vi "MEASURE_hysteresis_multiple_gate_Raman - set voltage.vi"() -> ()   [LabVIEW 2020]
uses:
  <instrlib>/Keithley 24XX/Public/Data/Read (Multiple Points).vi
  <vilib>/Utility/file.llb/Write To Spreadsheet File (DBL).vi
  <instrlib>/Stanford Research 830/Stanford Research 830.lvlib
  <instrlib>/Keithley 24XX/Keithley 24XX.lvlib
  <instrlib>/Keithley 2450/Keithley 2450.lvlib
  <vilib>/Analysis/NI_AALBase.lvlib
panel:
  in  "GATE final Value":dbl=6.0
  in  "Gate sequence":dbl
  out "while loop":dbl
  in  "topgate-off set":dbl=-5.0
  in  "0ff set{T}/no off set[F]":bool
  out "XY Graph 4":cluster{dbl[], dbl[]}(graph)
  out "XY Graph 3":cluster{dbl[], dbl[]}(graph)
  out "top gate leaking":dbl=2.469318360898143e-10
  out "bottom gate voltage":dbl format="%#_13g"
  in  "Compliance  Level (1uA)":dbl=1.9999999995789155e-07
  in  "Source Mode  (0: Voltage)":u16(ring) items=["Voltage", "Current"]
  in  "Serial Configuration":T1={"Baud Rate"=9600, "Parity"=0, "Data Bits"=8, "Stop Bits"=10, "Flow Control"=0} {"Flow Control" items=["None", "XON/XOFF", "RTS/CTS", "XON/XOFF & RTS/CTS", "DTR/DSR", "XON/XOFF & DTR/DSR"]; "Stop Bits" items=["1.0"=10, "1.5"=15, "2.0"=20]; "Data Bits" items=["7"=7, "8"=8]; "Parity" items=["None", "Odd", "Even", "Mark", "Space"]; "Baud Rate" items=["300"=300, "600"=600, "1200"=1200, "2400"=2400, "4800"=4800, "9600"=9600, "19200"=19200]}
  in  "backgate address":refnum<visa-resource-name>="GPIB0::25::INSTR"
  in  "bottom gate thickness":dbl=10.0
  in  "top gate thickness":dbl=30.0
  in  "pure field (T)/pure doping (F)":bool
  out "loop run":i32=2
  in  "loop #":i32=2
  in  "Save data or not":bool=TRUE
  in  "path (folder + filename)":string="C:\\Users\\User\\Data\\Jason\\03282019\\ pure_bottom_high_6v_rato3 with light2"
  in  "Clear Plot":bool
  out "LOCKIN Measurement":dbl=0.9110010000000001
  in  "Parameter (1: X)":u16(ring)=1 items=["X"=1, "Y"=2, "R"=3, "Theta"=4, "Channel 1"=5, "Channel 2"=6, "Aux In 1"=7, "Aux In 2"=8, "Aux In 3"=9, "Aux In 4"=10]
  out "top gate voltage":dbl format="%#_13g"
  out "back gate leaking":string="-9.306248E-12\n"
  in  "GATE STEP(mv)":i32=450
  in  "GATE Low Value (default 0)":dbl
  in  "GATE High Value":dbl=18.0
  in  "Function (0: Volts) 2":u16(ring) items=["Volts", "Current", "Resistance"]
  in  "Source Compaliance":dbl=1.000000000000001e-07
  in  "topgate address":refnum<visa-resource-name>="GPIB0::18::INSTR"
  in  "SD stabilization(S) 2":dbl=0.1 format="%#_13g"
  in  "Sine Output Amplitude (1 V) 2":dbl=0.05
  in  "GATE / SD stablization 3":dbl=0.1 format="%#_13g"
  in  "frequency":dbl=50.0 format="%#_13g"
  in  "Input Connection (0: Single-Ended Voltage)":u16(ring) items=["Single-Ended Voltage", "Differential Voltage", "1 MOhm Current Gain", "100 MOhm Current Gain"]
  in  "LOCKIN address":refnum<visa-resource-name>="GPIB0::8::INSTR"
  # "Gate2401(back) Setting"
  # "Lock-in"
  # "Gate2450(top) Setting"
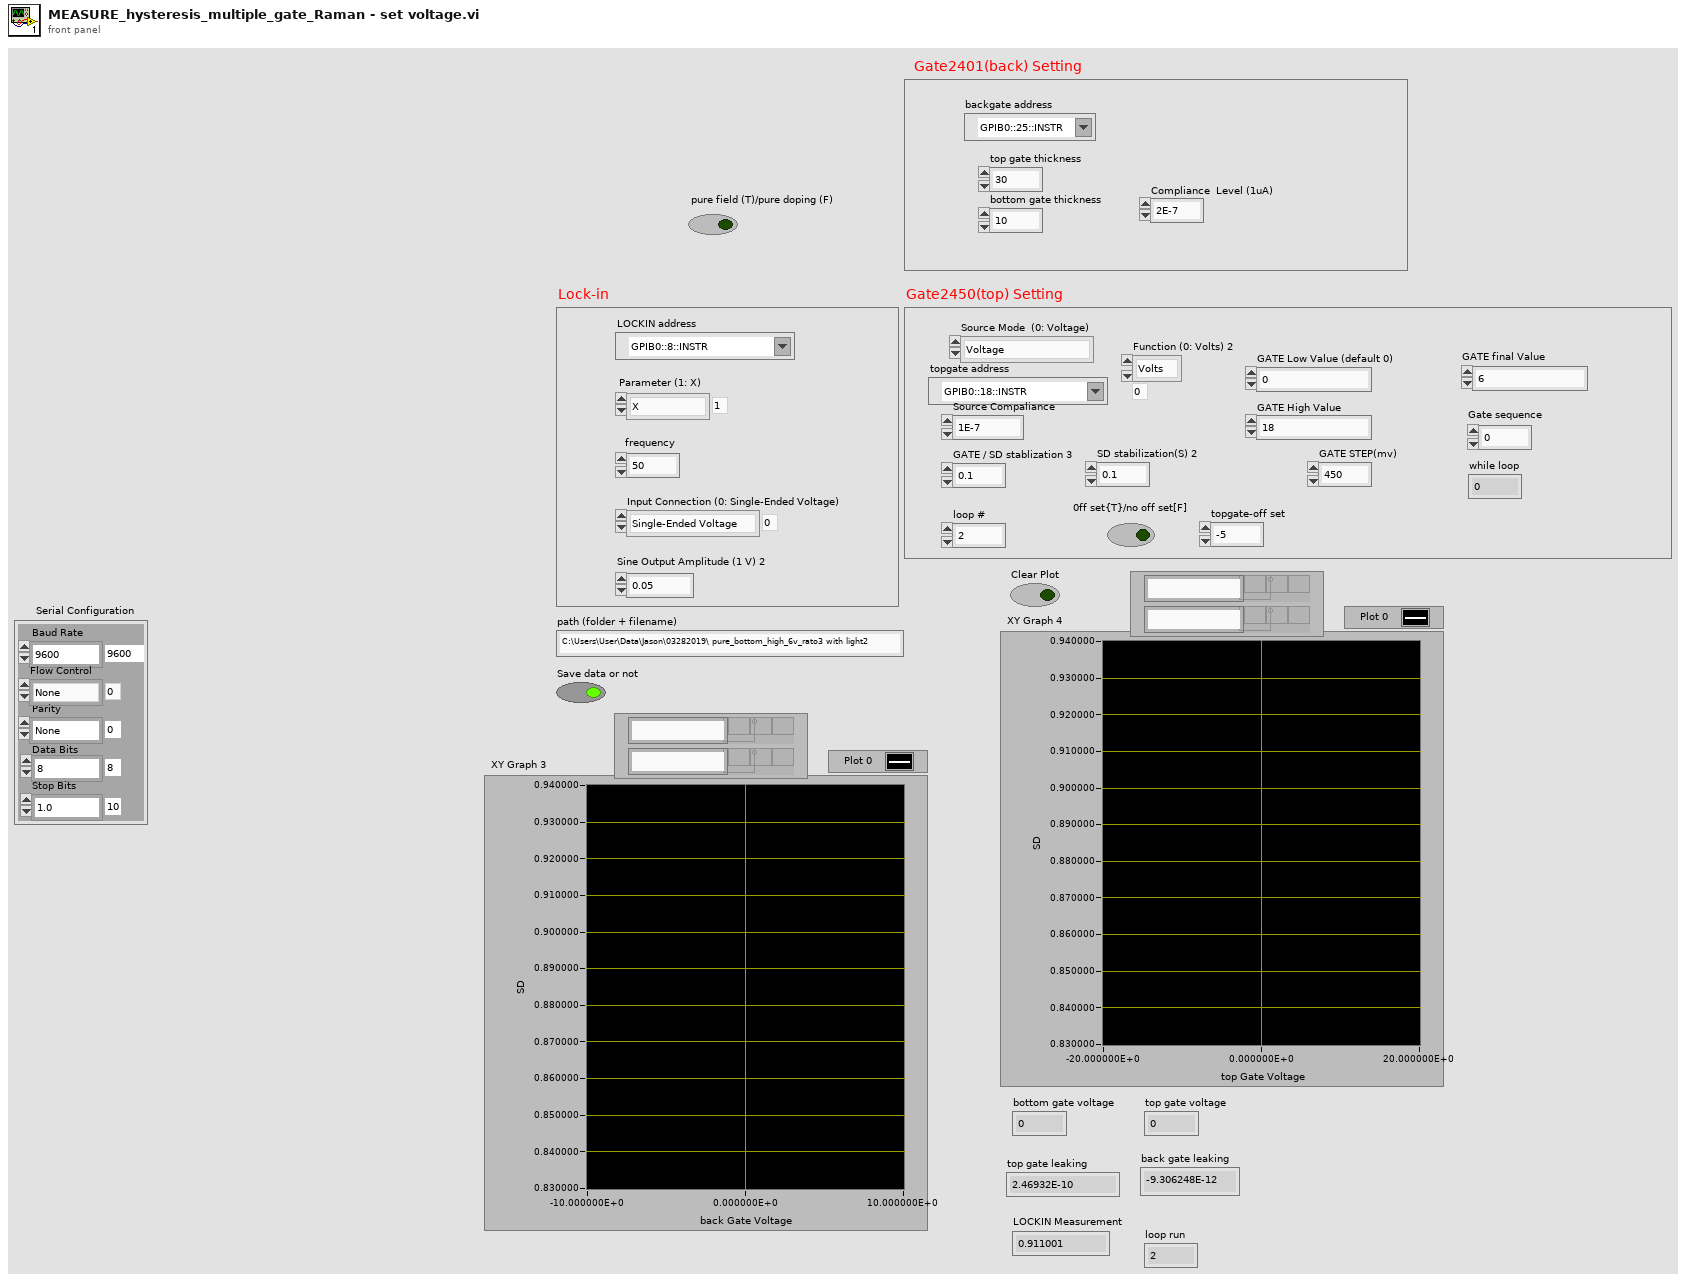
[diagram p1: front panel]
types:
  T1 = cluster{"Baud Rate":u32, "Parity":u16, "Data Bits":u16, "Stop Bits":u16, "Flow Control":u16}
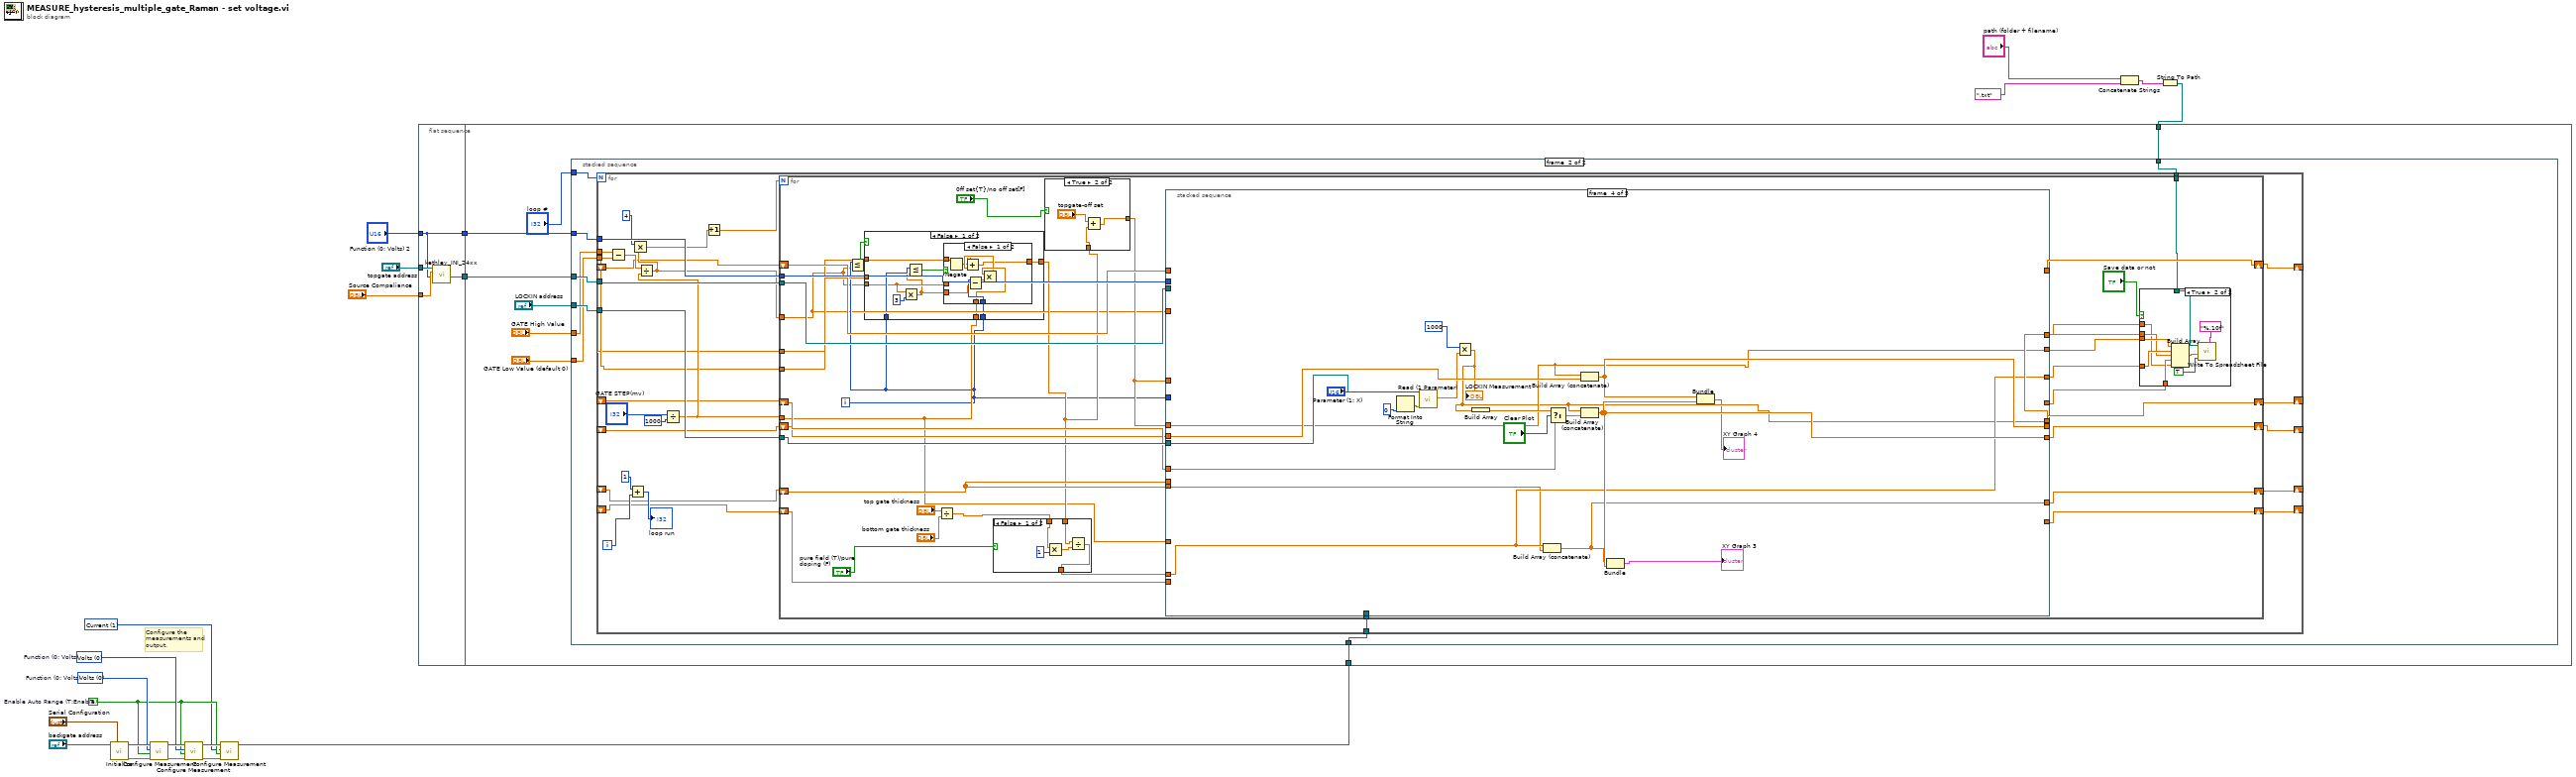
[diagram p0: block diagram]
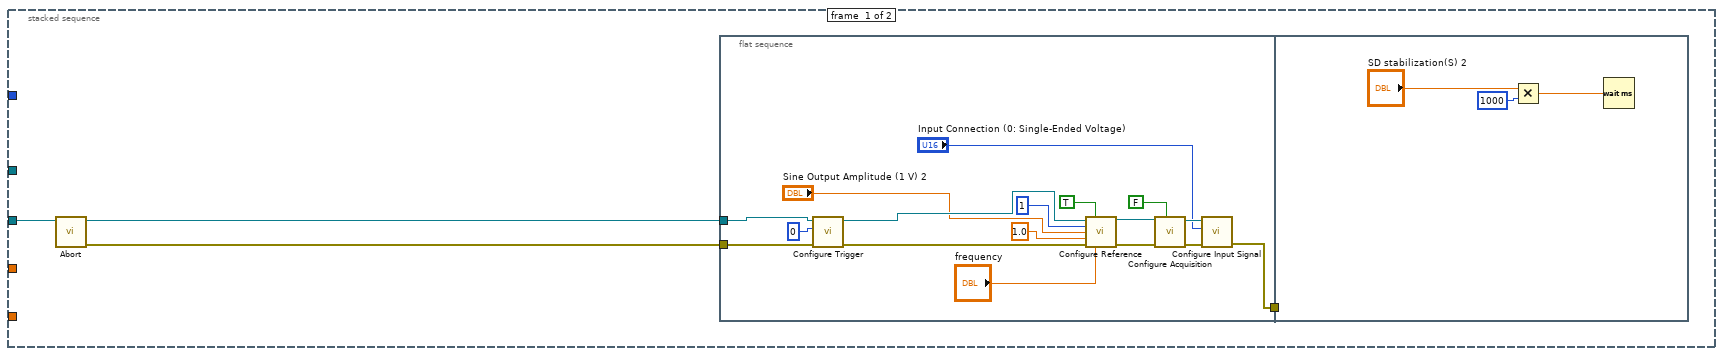
[diagram p2: hidden frame]
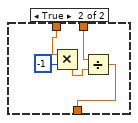
[diagram p4: hidden frame]
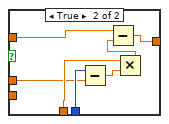
[diagram p6: hidden frame]
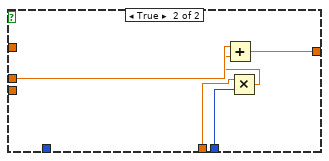
[diagram p7: hidden frame]
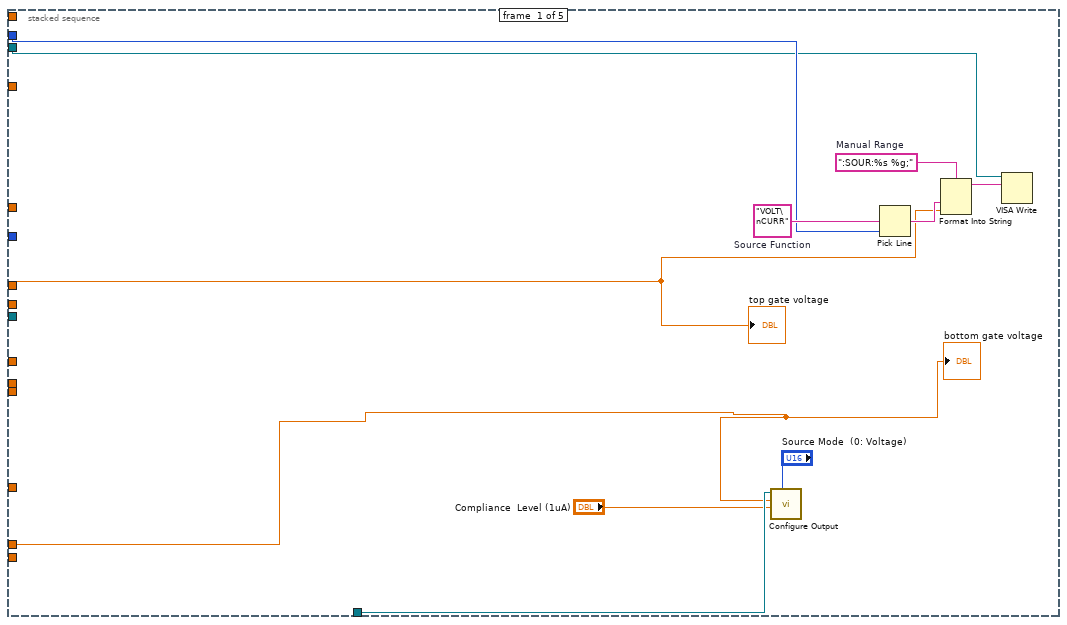
[diagram p8: hidden frame]
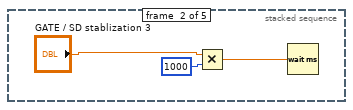
[diagram p9: hidden frame]
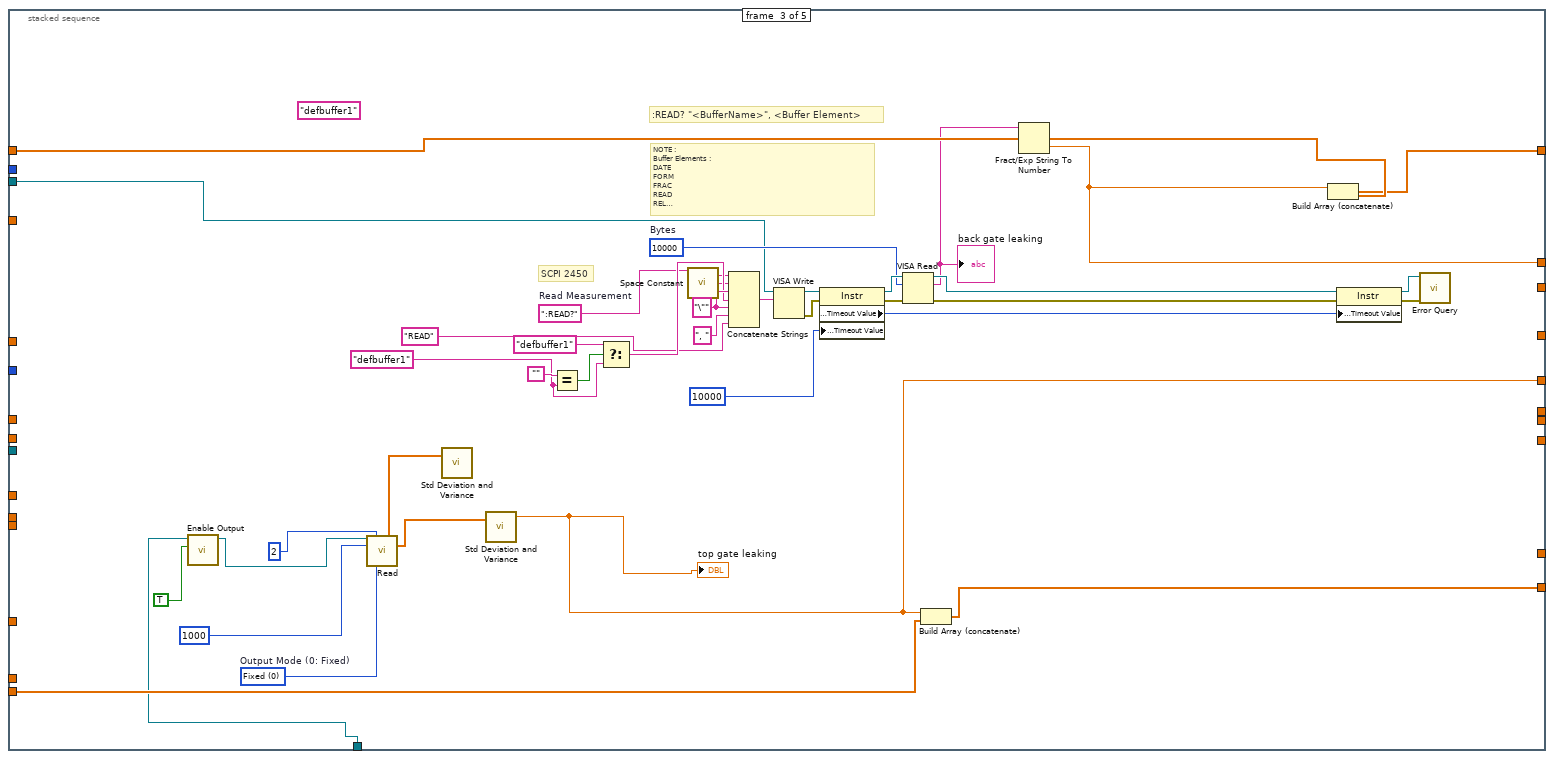
[diagram p10: hidden frame]
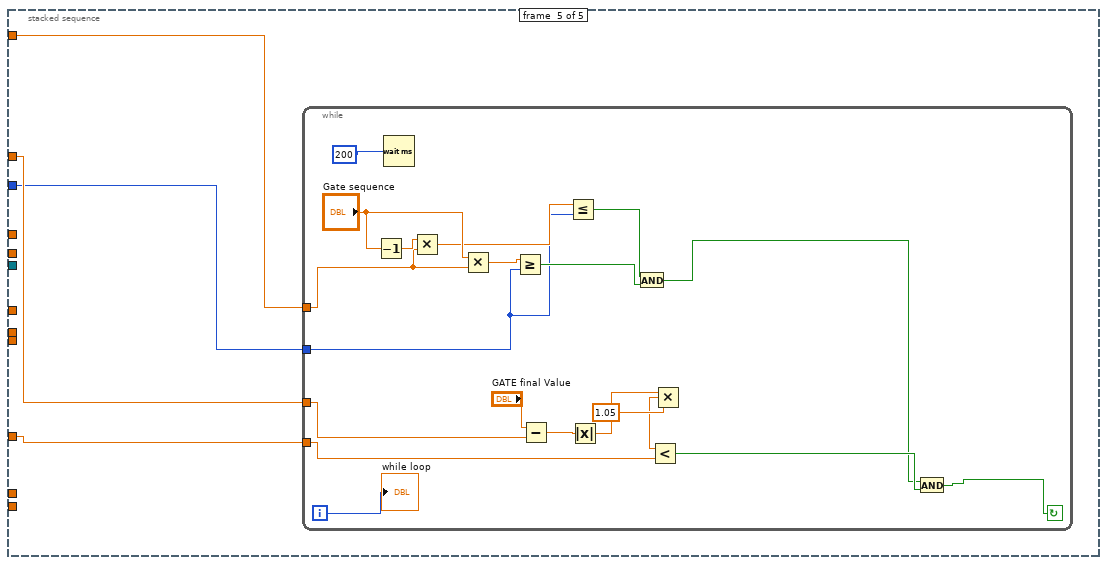
[diagram p11: hidden frame]
diagram:
  w2 = u16 1 items=["Volts", "Current", "Resistance"] ("Function (0: Volts)")
  w3 = TRUE  # Enable Auto Range (T:Enable)
  w6 = u16 0 items=["Volts", "Current", "Resistance"]  # Function (0: Volts)
  w7 = u16 0 items=["Volts", "Current", "Resistance"]  # Function (0: Volts)
  # "Configure the measurements and output."
  n1 = call <instrlib>:"Initialize.vi"("Serial Configuration"="Serial Configuration", "VISA resource name"="backgate address") -> ("error out"=w12:errorcluster, "VISA resource name out"=w13:refnum<visa-resource-name>)  [unwired: 8 in]
  n2 = call <instrlib>:"Configure Measurement.vi"("error in (no error)"=w12, "Enable Auto Range (T:Enable)"=w3, "Function (0: Volts)"=w7, "VISA resource name"=w13) -> ("error out"=w11:errorcluster, "VISA resource name out"=w10:refnum<visa-resource-name>)  [unwired: 6 in]
  n3 = call <instrlib>:"Configure Measurement.vi"("error in (no error)"=w11, "Enable Auto Range (T:Enable)"=w3, "Function (0: Volts)"=w6, "VISA resource name"=w10) -> ("error out"=w4:errorcluster, "VISA resource name out"=w5:refnum<visa-resource-name>)  [unwired: 6 in]
  n4 = call <instrlib>:"Configure Measurement.vi"("error in (no error)"=w4, "Enable Auto Range (T:Enable)"=w3, "Function (0: Volts)"=w2, "VISA resource name"=w5) -> ("VISA resource name out"=w1:refnum<visa-resource-name>)  [unwired: 6 in, 1 out]
  n5 = flat-sequence {
    tunnel: "topgate address" -> [w26]
    tunnel: "Source Compaliance" -> [w25]
    tunnel: "Function (0: Volts) 2" -> [w23]
    tunnel: [w24] -> w19
    tunnel: [w23] -> w18
    tunnel: w19 -> [w33]
    tunnel: w18 -> [w32]
    tunnel: w14 -> [w29]
    tunnel: w1 -> [w27]
    frame #0 {
      n6 = call "kethley_INI_24xx.vi"("Function (0: Volts) in"=w23, "Source Compaliance"=w25, "VISA Return in"=w26) -> ("VISA resource name out"=w24:refnum<visa-resource-name>)  [unwired: 8 in]
    }
    frame #1 {
      n7 = stacked-sequence {
        tunnel: "LOCKIN address" -> [w37 w64]
        tunnel: w33 -> [_ w65]
        tunnel: w32 -> [_ w66]
        tunnel: "GATE High Value" -> [_ w62]
        tunnel: "GATE Low Value (default 0)" -> [_ w63]
        tunnel: w29 -> [_ w61]
        tunnel: "loop #" -> [_ w60]
        tunnel: w27 -> [_ w59]
        frame #0 {
          n8 = call <instrlib>:"Abort.vi"("VISA resource name"=w37) -> ("error out"=w35:errorcluster, "VISA resource name out"=w36:refnum<visa-resource-name>)  [unwired: 9 in]
          n9 = flat-sequence {
            tunnel: w36 -> [w55]
            tunnel: [w40] -> w38
            tunnel: w35 -> [w39]
            tunnel: w38 -> [_]
            frame #0 {
              n10 = call <instrlib>:"Configure Trigger.vi"("error in (no error)"=w39, "Trigger Source (0: Internal)"=0, "VISA resource name"=w55) -> ("error out"=w49:errorcluster, "VISA resource name out"=w50:refnum<visa-resource-name>)  [unwired: 7 in]
              n11 = call <instrlib>:"Configure Reference.vi"("VISA resource name"=w50, "Auto Phase (T: Enabled)"=TRUE, "Reference Source (1: Internal)"=1, "Sine Output Amplitude (1 V)"="Sine Output Amplitude (1 V) 2", "Detection Harmonic Number (1)"=1.0 ("output voltage 2"), "error in (no error)"=w49, "Internal Reference Frequency (1000 Hz)"="frequency") -> ("VISA resource name out"=w47:refnum<visa-resource-name>, "error out"=w42:errorcluster)  [unwired: 7 in]
              n12 = call <instrlib>:"Configure Acquisition.vi"("Continuous Storage (T: Enable)"=FALSE, "error in (no error)"=w42, "VISA resource name"=w47) -> ("error out"=w41:errorcluster, "VISA resource name out"=w45:refnum<visa-resource-name>)  [unwired: 7 in]
              n13 = call <instrlib>:"Configure Input Signal.vi"("error in (no error)"=w41, "Input Connection (0: Single-Ended Voltage)"="Input Connection (0: Single-Ended Voltage)", "VISA resource name"=w45) -> ("error out"=w40:errorcluster)  [unwired: 7 in, 1 out]
            }
            frame #1 {
              n14 = Multiply(x="SD stabilization(S) 2", y=1000) -> (x*y=w58:dbl)
              n15 = Wait (ms)(milliseconds to wait=w58) -> ()  [unwired: 1 out]
            }
          }
        }
        frame #1 {
          n16 = for {
            N: w60 -> [_]
            tunnel: w66 -> [w94]
            tunnel: w65 -> [w93]
            tunnel: w64 -> [w92]
            tunnel: w63 -> [w86]
            tunnel: w62 -> [w85]
            tunnel: w61 -> [w84]
            shift-right: [w80] -> _
            shift-left: _ -> [w79]
            shift-right: [w78] -> _
            shift-left: _ -> [w76]
            shift-right: [w77] -> _
            shift-left: _ -> [w75]
            shift-right: [w71] -> _
            shift-left: _ -> [w70]
            shift-right: [w69] -> _
            shift-left: _ -> [w68]
            tunnel: w59 -> [w67]
            i -> [w73]
            n17 = Subtract(x=w85, y=w86) -> (x-y=w88:dbl)
            n18 = Add(x=1, y=w73) -> (x+y=→"loop run":i32)
            n19 = Divide(x="GATE STEP(mv)", y=1000) -> (x/y=w87:dbl)
            n20 = Divide(x=w88, y=w87) -> (x/y=w83:dbl)
            n21 = Multiply(x=4, y=w83) -> (x*y=w82:dbl)
            n22 = Increment(x=w82) -> (x+1=w81:dbl)
            n23 = for {
              N: w81 -> [_]
              tunnel: w94 -> [w129]
              tunnel: w93 -> [w128]
              tunnel: w92 -> [w127]
              tunnel: w87 -> [w97]
              shift-right: [w126] -> w80
              shift-left: w79 -> [w125]
              shift-right: [w122] -> w77
              shift-left: w75 -> [w124]
              shift-right: [w121] -> w78
              shift-left: w76 -> [w123]
              tunnel: w83 -> [w95]
              tunnel: w86 -> [w119]
              tunnel: w85 -> [w118]
              tunnel: w84 -> [w114]
              shift-right: [w112] -> w71
              shift-left: w70 -> [w103]
              shift-right: [w111] -> w69
              shift-left: w68 -> [w102]
              tunnel: w67 -> [w109]
              i -> [w96]
              n24 = Less Or Equal?(x=w96, y=w95) -> (x <= y?=w120:bool)
              n25 = case shown="False" w120 {
                tunnel: w119 -> [_ w181]
                tunnel: w96 -> [w161 w180]
                tunnel: w97 -> [w160 w179]
                tunnel: [w158 w177] -> w99
                tunnel: w118 -> [w159 _]
                tunnel: w95 -> [w154 _]
                tunnel: w96 -> [w157 _]
                frame False {
                  n26 = Multiply(x=w154, y=3) -> (x*y=w153:dbl)
                  n27 = Less Or Equal?(x=w157, y=w153) -> (x <= y?=w155:bool)
                  n28 = case shown="False" w155 {
                    tunnel: w161 -> [w169 w176]
                    tunnel: w160 -> [w167 w174]
                    tunnel: w159 -> [w163 w172]
                    tunnel: [w165 w171] -> w158
                    tunnel: w154 -> [_ w170]
                    tunnel: w153 -> [w162 _]
                    frame False {
                      n29 = Negate(x=w163) -> (-x=w164:dbl)
                      n30 = Subtract(x=w169, y=w162) -> (x-y=w168:dbl)
                      n31 = Multiply(x=w167, y=w168) -> (x*y=w166:dbl)
                      n32 = Add(x=w164, y=w166) -> (x+y=w165:dbl)
                    }
                    frame True {
                      n33 = Subtract(x=w176, y=w170) -> (x-y=w175:dbl)
                      n34 = Multiply(x=w174, y=w175) -> (x*y=w173:dbl)
                      n35 = Subtract(x=w172, y=w173) -> (x-y=w171:dbl)
                    }
                  }
                }
                frame True {
                  n36 = Multiply(x=w179, y=w180) -> (x*y=w178:dbl)
                  n37 = Add(x=w181, y=w178) -> (x+y=w177:dbl)
                }
              }
              n38 = Divide(x="top gate thickness", y="bottom gate thickness") -> (x/y=w108:dbl)
              n39 = case shown="False" "pure field (T)/pure doping (F)" {
                tunnel: w108 -> [w137 w143]
                tunnel: [w134 w141] -> w104
                tunnel: w99 -> [w135 w140]
                frame False {
                  n40 = Multiply(x=w137, y=1) -> (x*y=w136:dbl)
                  n41 = Divide(x=w135, y=w136) -> (x/y=w134:dbl)
                }
                frame True {
                  n42 = Multiply(x=w143, y=-1) -> (x*y=w139:dbl)
                  n43 = Divide(x=w140, y=w139) -> (x/y=w141:dbl)
                }
              }
              n44 = case shown="True" "0ff set{T}/no off set[F]" {
                tunnel: w99 -> [w130 w133]
                tunnel: [w130 w131] -> w98
                frame False {
                }
                frame True {
                  n45 = Add(x="topgate-off set", y=w133) -> (x+y=w131:dbl)
                }
              }
              n46 = stacked-sequence {
                tunnel: w129 -> [w188 _ _ _ _]
                tunnel: w128 -> [w187 _ w211 _ _]
                tunnel: w127 -> [_ _ _ w245 _]
                tunnel: w98 -> [w186 _ _ w244 _]
                tunnel: [_ _ w209 _ _] -> w126
                tunnel: w125 -> [_ _ w210 _ _]
                tunnel: w124 -> [_ _ _ w248 _]
                tunnel: w123 -> [_ _ _ w246 _]
                tunnel: [_ _ _ w241 _] -> w122
                tunnel: [_ _ _ w247 _] -> w121
                tunnel: [_ _ _ w235 _] -> w117
                tunnel: [_ _ _ w244 _] -> w116
                tunnel: [_ _ w207 _ _] -> w115
                tunnel: [_ _ w201 _ _] -> w112
                tunnel: [_ _ _ w240 _] -> w111
                tunnel: w102 -> [_ _ _ _ _]
                tunnel: [_ _ _ w239 _] -> w110
                tunnel: [_ _ w200 _ _] -> w101
                tunnel: w109 -> [w184 _ w197 _ _]
                tunnel: w104 -> [w182 _ _ w239 _]
                tunnel: w103 -> [_ _ w199 _ _]
                tunnel: w102 -> [_ _ _ w238 _]
                tunnel: w98 -> [_ _ _ _ w257]
                tunnel: w97 -> [_ _ _ _ w256]
                tunnel: w96 -> [_ _ _ _ w255]
                tunnel: w95 -> [_ _ _ _ w254]
                frame #0 {
                  w190 = "VOLT\nCURR"  # Source Function
                  w191 = ":SOUR:%s %g;"  # Manual Range
                  n47 = call <instrlib>:"Configure Output.vi"("Source Mode  (0: Voltage)"="Source Mode  (0: Voltage)", "Compliance  Level (0.1)"="Compliance  Level (1uA)", "Output Level (0)"=w182, "VISA resource name"=w184) -> ()  [unwired: 6 in, 2 out]
                  n48 = Pick Line(multi-line string=w190, line index=w188) -> (output string=w189:string)  [unwired: 1 out]
                  n49 = Format Into String(format string=w191, w189, w186) -> (resulting string=w192:string)  [unwired: 2 in, 1 out]
                  n50 = VISA Write(VISA resource name=w187, write buffer=w192) -> ()  [unwired: 1 in, 3 out]
                  "top gate voltage" <- w186
                  "bottom gate voltage" <- w182
                }
                frame #1 {
                  n51 = Multiply(x="GATE / SD stablization 3", y=1000) -> (x*y=w195:dbl)
                  n52 = Wait (ms)(milliseconds to wait=w195) -> ()  [unwired: 1 out]
                }
                frame #2 {
                  w204 = u16 0 items=["Fixed", "Sweep", "List"]  # Output Mode (0: Fixed)
                  w222 = "defbuffer1" ("Buffer Name (defbuffer1) 2")
                  (unwired) "defbuffer1" ("t")
                  w220 = "\""
                  w217 = ":READ?"  # Read Measurement
                  w226 = u32 10000  # Bytes
                  # "NOTE :\nBuffer Elements :\nDATE\nFORM\nFRAC\nREAD\nREL\nSEC\nSOUR\nSOURFORM\nSOURSTAT\nSOURUNIT\nSTAT\nTIME\nTsT\nUNIT"
                  # ":READ? \"<BufferName>\", <Buffer Element>"
                  # "SCPI 2450"
                  n53 = call <instrlib>:"Enable Output.vi"("Enable Output (T: Enable)"=TRUE, "VISA resource name"=w197) -> ("VISA resource name out"=w196:refnum<visa-resource-name>)  [unwired: 8 in, 1 out]
                  n54 = call-poly <instrlib>:"Read.vi"("VISA resource name"=w196, "Sample Count (1)"=u32 2 ("Number of Samples"), "Timeout (10000 ms)"=1000, "Output Mode (0: Fixed)"=w204) -> ("Voltage"=w202:sgl[], "Current"=w203:sgl[])  [unwired: 5 in, 5 out]
                  n55 = call <vilib>:"Std Deviation and Variance.vi"("X"=w202) -> ()  [unwired: 1 in, 3 out]
                  n56 = call <vilib>:"Std Deviation and Variance.vi"("X"=w203) -> ("mean"=w200:dbl)  [unwired: 1 in, 2 out]
                  "top gate leaking" <- w200
                  n57 = Equal?(x="", y=w222) -> (x = y?=w223:bool)
                  n58 = Select(t="defbuffer1", s=w223, f=w222) -> (s? t:f=w219:string)
                  n59 = call <vilib>:"Space Constant.vi"() -> ("String"=w218:string)
                  n60 = Concatenate Strings(w217, w218, w220, w219, w220, ", " ("string"), "READ" ("Buffer Elements 2")) -> (w233:string)
                  n61 = VISA Write(VISA resource name=w211, write buffer=w233) -> (VISA resource name out=w225:refnum<visa-resource-name>, error out=w232:errorcluster)  [unwired: 1 in, 1 out]
                  n62 = property class="Instr"(reference=w225, error in=w232, "General Settings:Timeout Value"=10000 ("Timeout (10000 ms) 2")) -> (reference out=w231:refnum<visa-resource-name>, error out=w230:errorcluster, "General Settings:Timeout Value"=w227:u32)
                  n63 = VISA Read(VISA resource name=w231, byte count=w226, error in (no error)=w230) -> (VISA resource name out=w229:refnum<visa-resource-name>, read buffer=w208:string, error out=w228:errorcluster)  [unwired: 1 out]
                  "back gate leaking" <- w208
                  n64 = Build Array (concatenate)(w200, w199) -> (w201:dbl[])
                  n65 = Fract/Exp String To Number(string=w208) -> (number=w207:dbl)  [unwired: 3 in, 1 out]
                  n66 = Build Array (concatenate)(w207, w210) -> (w209:dbl[])
                  n67 = property class="Instr"(reference=w229, error in=w228, "General Settings:Timeout Value"=w227) -> (reference out=w215:refnum<visa-resource-name>, error out=w214:errorcluster)
                  n68 = call <instrlib>:"Error Query.vi"("error in (no error)"=w214, "VISA resource name"=w215) -> ()  [unwired: 10 out]
                }
                frame #3 {
                  n69 = Format Into String(0) -> (error out=w253:errorcluster)  [unwired: 3 in, 1 out]
                  n70 = call <instrlib>:"Read (1 Parameter).vi"("error in (no error)"=w253, "Parameter (1: X)"="Parameter (1: X)", "VISA resource name"=w245) -> ("Measurement"=w236:dbl)  [unwired: 6 in, 2 out]
                  n71 = Multiply(x=1000, y=w236) -> (x*y=w235:dbl)
                  "LOCKIN Measurement" <- w235
                  n72 = Build Array(w235) -> (w251:dbl[])
                  n73 = Build Array (concatenate)(w239, w238) -> (w240:dbl[])
                  n74 = Select(t=w251, s="Clear Plot", f=w248) -> (s? t:f=w243:dbl[])
                  n75 = Build Array (concatenate)(w244, w246) -> (w247:dbl[])
                  n76 = Build Array (concatenate)(w235, w243) -> (w241:dbl[])
                  n77 = Bundle(w240, w241) -> (→"XY Graph 3":cluster{dbl[], dbl[]})  [unwired: 1 in]
                  n78 = Bundle(w247, w241) -> (→"XY Graph 4":cluster{dbl[], dbl[]})  [unwired: 1 in]
                }
                frame #4 {
                  n79 = while {
                    tunnel: w255 -> [w263]
                    tunnel: w254 -> [w267]
                    tunnel: w256 -> [w272]
                    tunnel: w257 -> [w270]
                    i -> [w277]
                    stop <- w275 continue-if-true
                    n80 = Decrement(x="Gate sequence") -> (x-1=w268:dbl)
                    n81 = Wait (ms)(milliseconds to wait=200) -> ()  [unwired: 1 out]
                    n82 = Multiply(x=w268, y=w267) -> (x*y=w264:dbl)
                    n83 = Multiply(x="Gate sequence", y=w267) -> (x*y=w266:dbl)
                    n84 = Greater Or Equal?(x=w266, y=w263) -> (x >= y?=w265:bool)
                    n85 = Subtract(x="GATE final Value", y=w270) -> (x-y=w273:dbl)
                    n86 = Less Or Equal?(x=w264, y=w263) -> (x <= y?=w262:bool)
                    n87 = Absolute Value(x=w273) -> (abs(x)=w260:dbl)
                    n88 = And(x=w262, y=w265) -> (x .and. y?=w261:bool)
                    n89 = Multiply(x=w260, y=1.05) -> (x*y=w258:dbl)
                    n90 = Less?(x=w258, y=w272) -> (x < y?=w271:bool)
                    n91 = And(x=w261, y=w271) -> (x .and. y?=w275:bool)
                    "while loop" <- w277
                  }
                }
              }
              n92 = case shown="True" "Save data or not" {
                tunnel: w117 -> [_ w145]
                tunnel: w116 -> [_ w152]
                tunnel: w115 -> [_ w144]
                tunnel: w114 -> [_ w150]
                tunnel: w110 -> [_ w146]
                tunnel: w101 -> [_ w147]
                frame False {
                }
                frame True {
                  n93 = Build Array(w152, w146, w145, w147, w144) -> (w151:dbl[])
                  n94 = call-poly <vilib>:"Write To Spreadsheet File.vi"("format (%.3f)"="%.10f", "append to file? (new file:F)"=TRUE, "1D data"=w151, "file path (dialog if empty)"=w150) -> ()  [unwired: 4 in, 1 out]
                }
              }
            }
          }
        }
      }
    }
  }
  n95 = Concatenate Strings("path (folder + filename)", ".txt") -> (w15:string)
  n96 = String To Path(string=w15) -> (path=w14:path)
